vi "Nearest.vi"(10 "Target":dbl[](array[numeric]), 11 "Pontos":dbl[][](array[numeric])) -> (2 "Nearest":dbl[](array[numeric]))   [LabVIEW 2018]
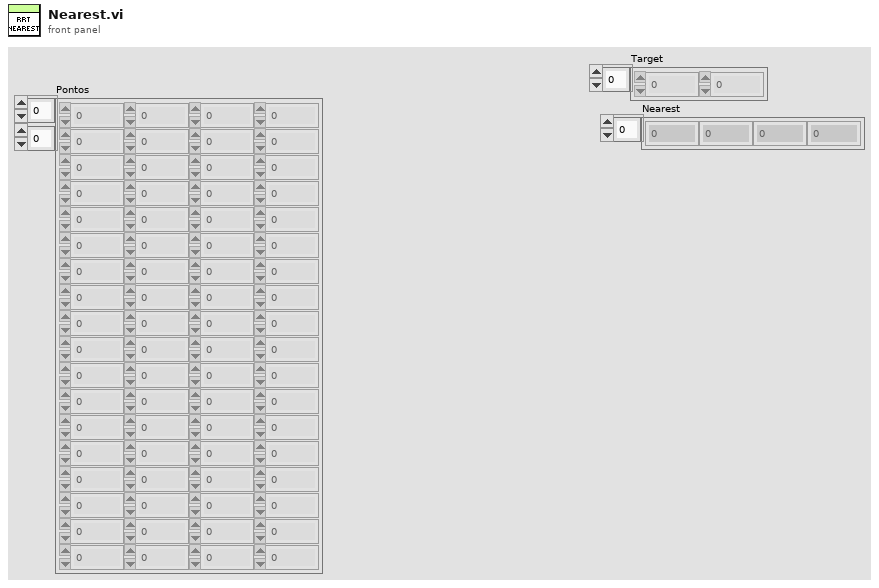
[diagram p1: front panel]
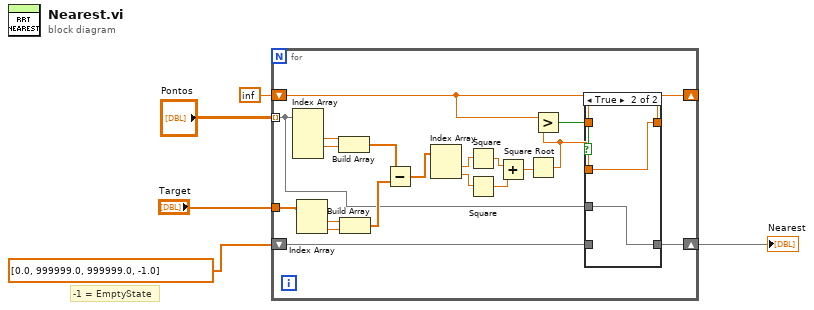
[diagram p0: block diagram]
diagram:
  # "-1 = EmptyState"
  n1 = for {
    tunnel: "Pontos" -> [w16] mode=indexing
    shift-right: [w20] -> _
    shift-left: inf -> [w19]
    tunnel: "Target" -> [w15]
    shift-right: [w13] -> w1
    shift-left: dbl[] [0.0, 999999.0, 999999.0, -1.0] ("Nearest 2") -> [w14]
    n2 = Index Array(array=w16) -> (element #2=w25:dbl, element #3=w24:dbl)  [unwired: 4 in, 2 out]
    n3 = Index Array(array=w15) -> (element #1=w18:dbl, element #2=w17:dbl)  [unwired: 2 in]
    n4 = Build Array(w25, w24) -> (w23:dbl[])
    n5 = Build Array(w18, w17) -> (w22:dbl[])
    n6 = Subtract(x=w23, y=w22) -> (x-y=w12:dbl[])
    n7 = Index Array(array=w12) -> (element #1=w11:dbl, element #2=w10:dbl)  [unwired: 2 in]
    n8 = Square(x=w11) -> (x^2=w9:dbl)
    n9 = Square(x=w10) -> (x^2=w8:dbl)
    n10 = Add(x=w9, y=w8) -> (x+y=w7:dbl)
    n11 = Square Root(x=w7) -> (sqrt(x)=w6:dbl)
    n12 = Greater?(x=w19, y=w6) -> (0:w21:bool)
    n13 = case shown="True" w21 {
      tunnel: [w27 w28] -> w20
      tunnel: w19 -> [w27 _]
      tunnel: w16 -> [_ w29]
      tunnel: [w26 w29] -> w13
      tunnel: w14 -> [w26 _]
      tunnel: w6 -> [_ w28]
      frame False {
      }
      frame True {
      }
    }
  }
  "Nearest" <- w1
